vi "Actor Core.vi"(8 "error in":errorcluster, 11 "TranslationStageUI.lvclass":refnum<class "TranslationStageUI.lvclass">) -> (0 "error out":errorcluster, 3 "Actor out":refnum<class "Actor.lvclass">)   [LabVIEW 2023, in "TranslationStage_UI.lvlib" / "TranslationStageUI.lvclass"]
doc: "(<B>Filename</B>: Actor Framework.lvlib:Actor.lvclass:Actor Core.vi)\n\nReceives messages to the actor, reacts to them, and initiates any error handling that may shut the actor down.\n\nDescendant classes may override this VI to append parallel tasks for the actor to complete while it handles messages. Overrides use the Call Parent Class Method node."
uses:
  TranslationStageUI.lvclass
  <vilib>/ActorFramework/Actor/Actor.lvclass
  Scan_Data_For_Controller.ctl
  typedefs/TranslationStagePublicData.ctl
  <vilib>/ActorFramework/Actor/Actor.lvclass/Actor.ctl
  <vilib>/ActorFramework/Message Enqueuer/Message Enqueuer.lvclass/Message Enqueuer.ctl
  TranslationStageUI.lvclass/TranslationStageUI.ctl
  ConcreteClasses/ConcreteInstrumentClasses/KIM101/KIM101/KIM101.lvclass
  ConcreteClasses/ConcreteInstrumentClasses/Jiaxin_Stepper_Controller/Jiaxin_Stepper_Controller/Jiaxin_Stepper_Controller.lvclass
  Interfaces/InitDeinitInterface/InitDeinit Messages/Init Msg/Init Msg.lvclass/Init Msg.ctl
  Interfaces/AbstractInstrumentClasses/TranslationStages_LV/TranslationStagesInterface Messages/Goto Msg/Goto Msg.lvclass/Goto Msg.ctl
  Interfaces/AbstractInstrumentClasses/TranslationStages_LV/TranslationStagesInterface Messages/MoveBySteps Msg/MoveBySteps Msg.lvclass/MoveBySteps Msg.ctl
  SinglePhotonUI/Libraries/SPIController/SPIController Messages/InitScan Msg/InitScan Msg.lvclass/InitScan Msg.ctl
  SinglePhotonUI/Libraries/SPIController/SPIController Messages/StageMoved Msg/StageMoved Msg.lvclass/StageMoved Msg.ctl
  ConcreteClasses/ConcreteInstrumentClasses/Jiaxin_Stepper_Controller/Jiaxin_Stepper_Controller Messages/JX_GoHome Msg/JX_GoHome Msg.lvclass/JX_GoHome Msg.ctl
  <vilib>/ActorFramework/Message Enqueuer/Init from Existing Queue.vi
  <vilib>/ActorFramework/Message Enqueuer/Enqueue.vi
  Interfaces/InitDeinitInterface/InitDeinit Messages/Init Msg/Init Msg.lvclass
  <vilib>/ActorFramework/Stop Msg/Stop Msg.lvclass
  Interfaces/AbstractInstrumentClasses/TranslationStages_LV/TranslationStagesInterface Messages/Goto Msg/Goto Msg.lvclass
  Interfaces/AbstractInstrumentClasses/TranslationStages_LV/TranslationStagesInterface Messages/MoveBySteps Msg/MoveBySteps Msg.lvclass
  ConcreteClasses/ConcreteInstrumentClasses/Jiaxin_Stepper_Controller/Jiaxin_Stepper_Controller Messages/JX_SetHome Msg/JX_SetHome Msg.lvclass
  SinglePhotonUI/Libraries/SPIController/SPIController Messages/InitScan Msg/InitScan Msg.lvclass
  SinglePhotonUI/Libraries/SPIController/SPIController Messages/StageMoved Msg/StageMoved Msg.lvclass
  ConcreteClasses/ConcreteInstrumentClasses/Jiaxin_Stepper_Controller/Jiaxin_Stepper_Controller Messages/JX_GoHome Msg/JX_GoHome Msg.lvclass
  <vilib>/ActorFramework/Message Priority Queue/Priority Enqueue.vi
  <vilib>/ActorFramework/Message Enqueuer/Message Enqueuer.lvclass
  SinglePhotonUI/Libraries/SinglePhotonInterferenceUI/SinglePhotonInterferenceUI/SinglePhotonInterferenceUI.lvclass
  typedefs/typedefs.lvlib
  C:/Program Files/National Instruments/LabVIEW 2023/vi.lib/ActorFramework/Actor/Actor.lvclass
  C:/Users/quantum/Documents/LVDAQ/UIs/TranslationStage_UI/TranslationStage_UI/TranslationStageUI.lvclass
  C:/Users/quantum/Documents/LVDAQ/Interfaces/InitDeinitInterface/InitDeinitComm/InitDeinitComm.lvclass
  C:/Users/quantum/Documents/LVDAQ/Interfaces/AbstractInstrumentClasses/TranslationStages_LV/TranslationStagesComm/TranslationStagesComm.lvclass
  <vilib>/Utility/Data Type/NI_Data Type.lvlib
panel:
  out "value":variant
  in  "Go To":bool
  in  "Tab Control":T1(tab)
  in  "VISA resource name":refnum<visa-resource-name>
  in  "Control":enum16{"KIM", "Stepper Motors"}(ring)=enum."Stepper Motors"
  in  "Address":string="97102699"
  in  "Init motor":bool
  in  "Restart Piezo":bool
  in  "Exit":bool
  in  "Experiment Jog":i32(ring) caption="Experiment" items=["Imaging", "Interferometer"]
  in  "Jog Left HOM":bool
  in  "Jog Right HOM":bool
  in  "Jog Up":bool
  in  "Jog Left":bool
  in  "Jog Right":bool
  in  "Jog Down":bool
  in  "Jog Z Out":bool
  in  "Jog Z In":bool
  in  "Steps":i32(slide)=1 min=1 max=60000 step=1 scale=1.0..60000.0
  out "Position X":i32
  out "Position Z":i32
  out "Position Y":i32
  out "Position HOM":i32
  out "Scanning":bool
  in  "Get Measurements":bool
  in  "Steps Per Segment":i32=1 min=1 max=60000 step=1
  in  "Interferometer\nDirection":enum16{"Forward", "Backwards"}(ring)=enum."Backwards"
  in  "Focus Scan Direction":enum16{"Forward", "Backwards"}(ring)=enum."Backwards"
  in  "Y Scan Direction":enum16{"Forward", "Backwards"}(ring)=enum."Backwards"
  in  "Focus Steps":u32=1 min=1 max=60000 step=1
  in  "Y Pixels":u32=1 min=1 max=60000 step=1
  in  "X Pixels":u32=1 min=1 max=60000 step=1
  in  "Scan":bool
  in  "Acq Per Step":u8=1 min=1 step=1
  in  "X Scan Direction":enum16{"Forward", "Backwards"}(ring)=enum."Backwards"
  in  "Interferometer\nSegments":u32=1 min=1 max=60000 step=1
  in  "Experiment Scan":i32(ring) caption="Experiment" items=["Imaging", "Interferometer"]
  in  "HOM Channel":i32(ring)=1 items=["Channel0", "Channel1", "Channel2", "Channel3", "Channel4"]
  in  "Z Channel":i32(ring)=1 items=["Channel0", "Channel1", "Channel2", "Channel3", "Channel4"]
  in  "Y Channel":i32(ring)=1 items=["Channel0", "Channel1", "Channel2", "Channel3", "Channel4"]
  in  "X Channel":i32(ring)=1 items=["Channel0", "Channel1", "Channel2", "Channel3", "Channel4"]
  in  "Scan Data":T2
  in  "Scan Data":T2
  out "VI":refnum<vi>
  in  "Jog Parameters":T3={"JogAcceleration"=0, "JogStepFwd"=1, "JogMode"=1, "JogRate"=0, "JogStepRev"=1} {"JogStepRev" min=1 max=50000 step=1; "JogMode" items=["Continuous"=1, "Step"=2]; "JogStepFwd" min=1 max=100000 step=1}
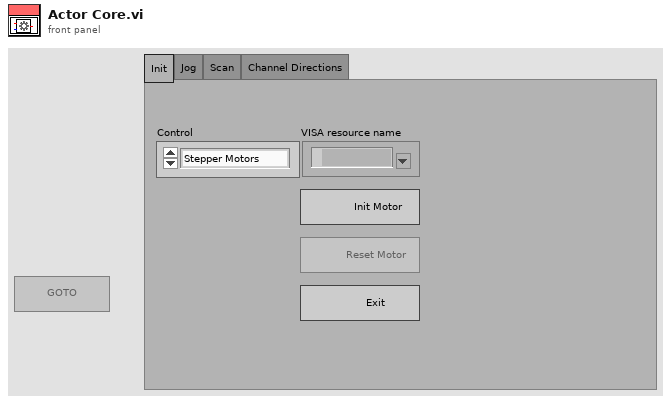
[diagram p1: front panel]
types:
  T1 = enum32{"Init", "Jog", "Scan", "Channel Directions"}
  T2 = typedef "typedefs.lvlib/Scan_Data_For_Controller.ctl" = cluster{"Scan Segments X":u32, "Scan Segments Y":u32, "Acq per step":u8, "Get Measurements?":bool}
  T3 = cluster{"JogAcceleration":i32, "JogStepFwd":i32, "JogMode":i32, "JogRate":i32, "JogStepRev":i32}
  T4 = typedef "typedefs.lvlib/TranslationStagePublicData.ctl" = cluster{"Scanning Instrument":bool, "Path":path, "FileName":string, "Scan Segments":u32, "Step Time (us)":u32, "Polarity":enum16{"Positive", "Negative"}, "Direction":enum16{"Forward", "Backwards"}, "Steps":u32, "Acq per step":u32, "First Scan Move?":bool, "Scan Segments X":u32, "Scan Segments Y":u32, "Position":i32, "Position 2":i32, "Position 3":i32, "Position 4":i32, "Home 1":i32, "Home 2":i32, "Home 3":i32, "Home 4":i32, "Going Home?":bool, "Selected Motor":enum16{"KIM", "Stepper Motors"}, "Scanning Motor":bool}
  T5 = enum8{"Enabled", "Disabled", "Disabled and Grayed Out"}
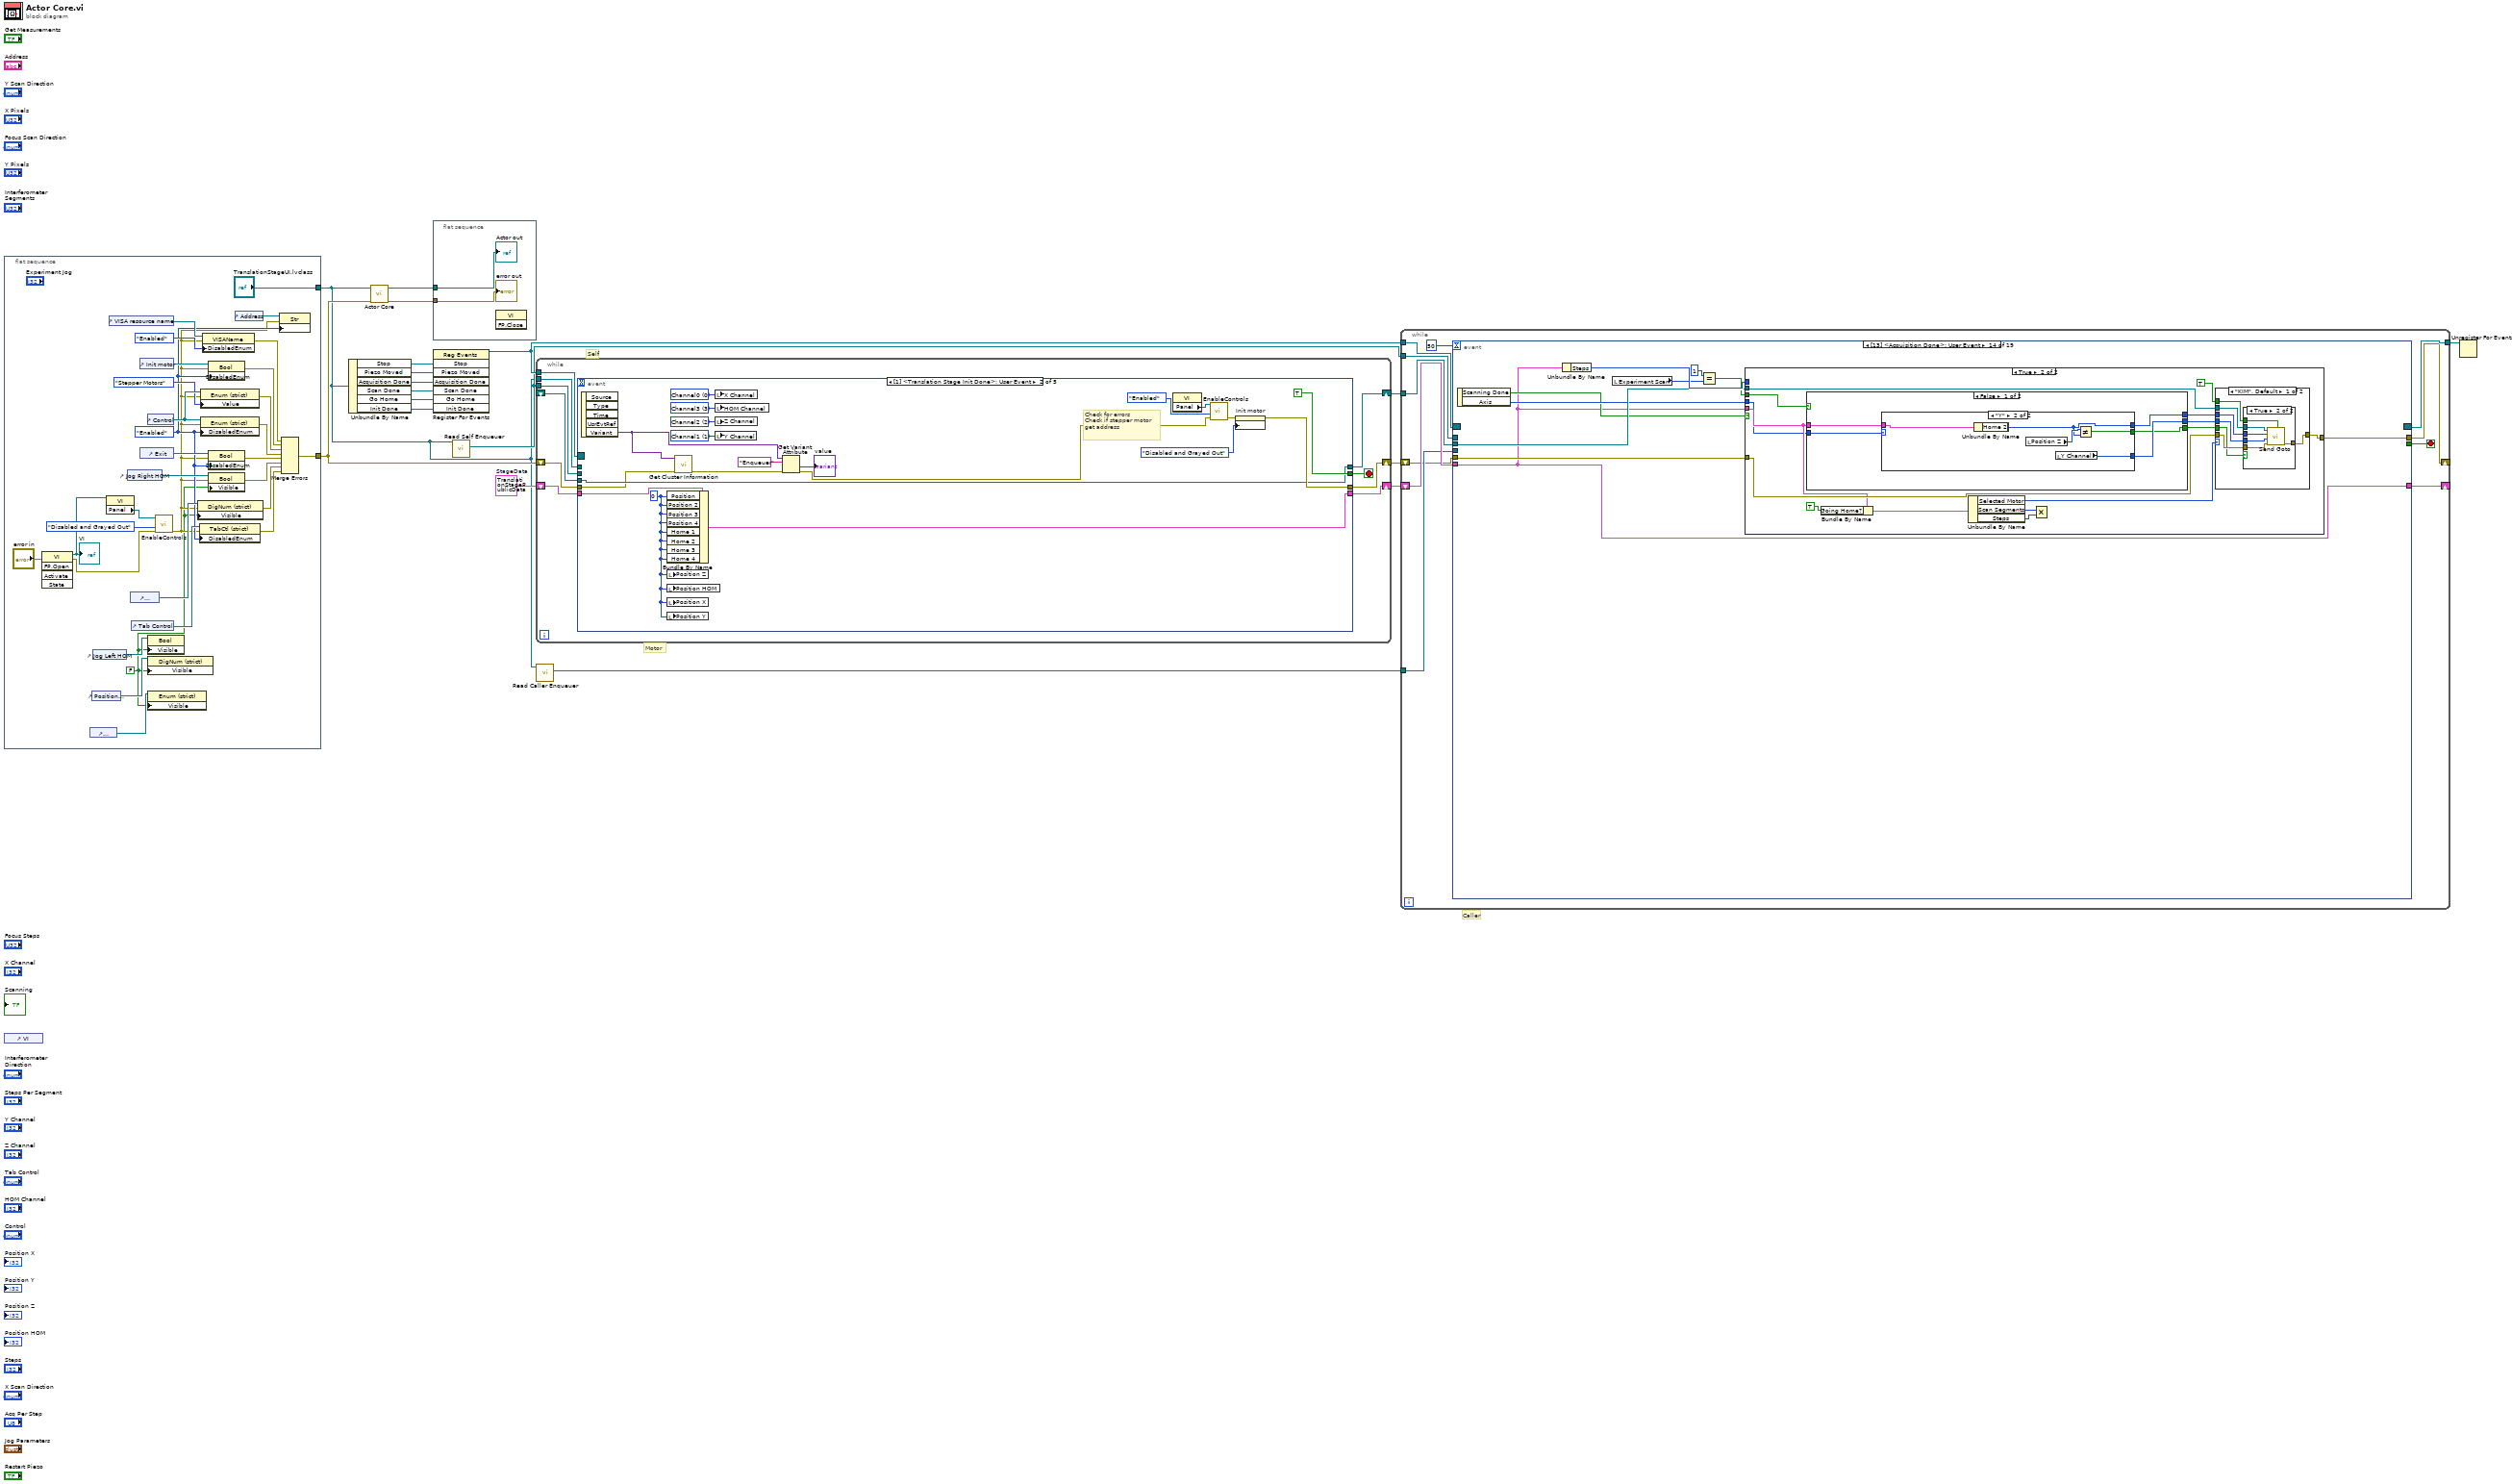
[diagram p0: block diagram]
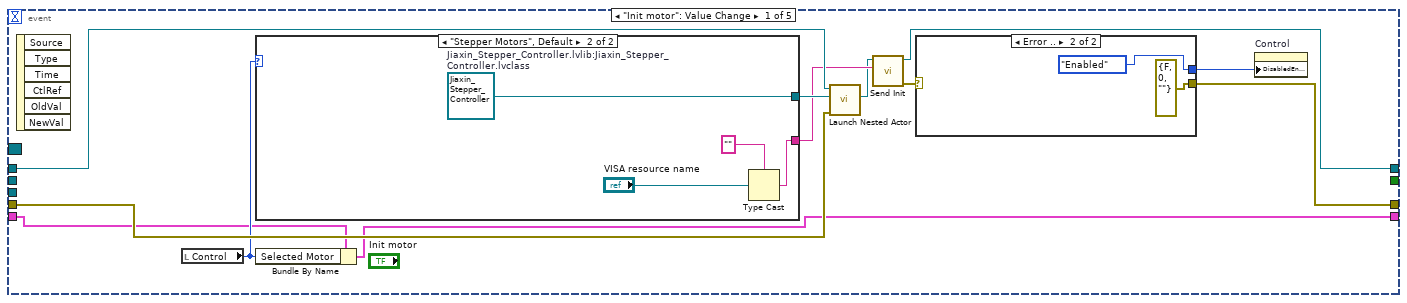
[diagram p2: hidden frame]
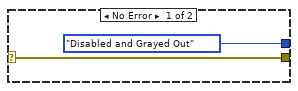
[diagram p3: hidden frame]
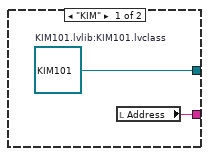
[diagram p4: hidden frame]
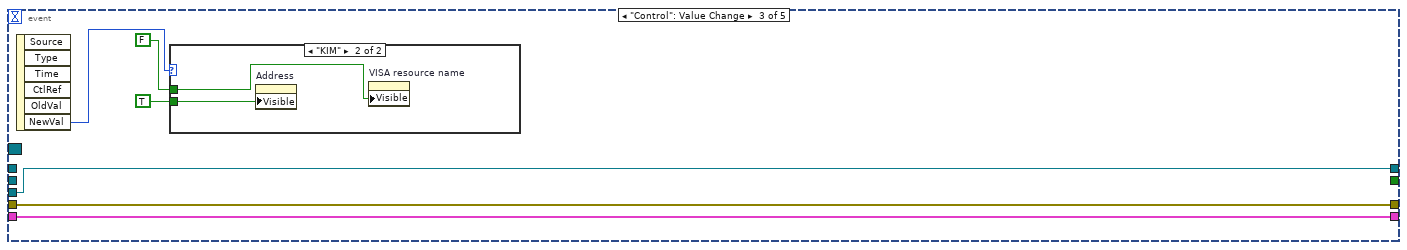
[diagram p5: hidden frame]
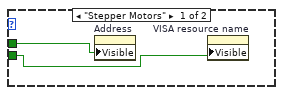
[diagram p6: hidden frame]
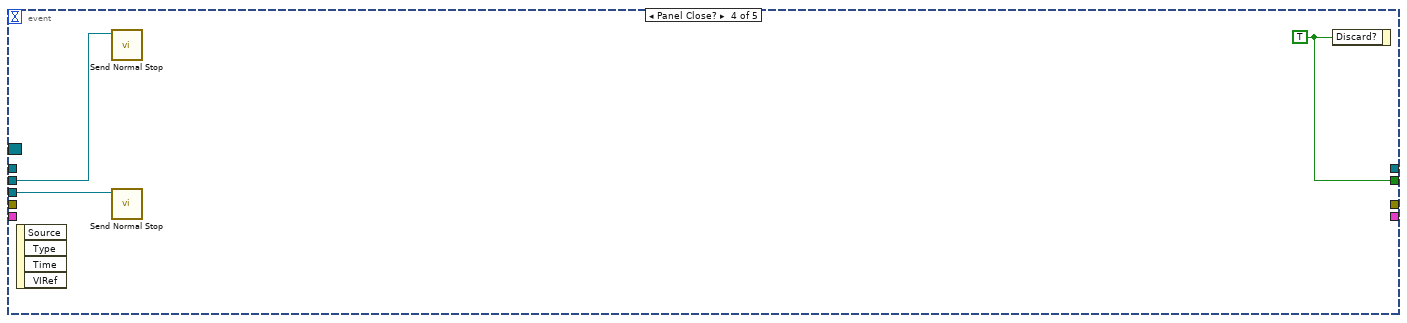
[diagram p7: hidden frame]
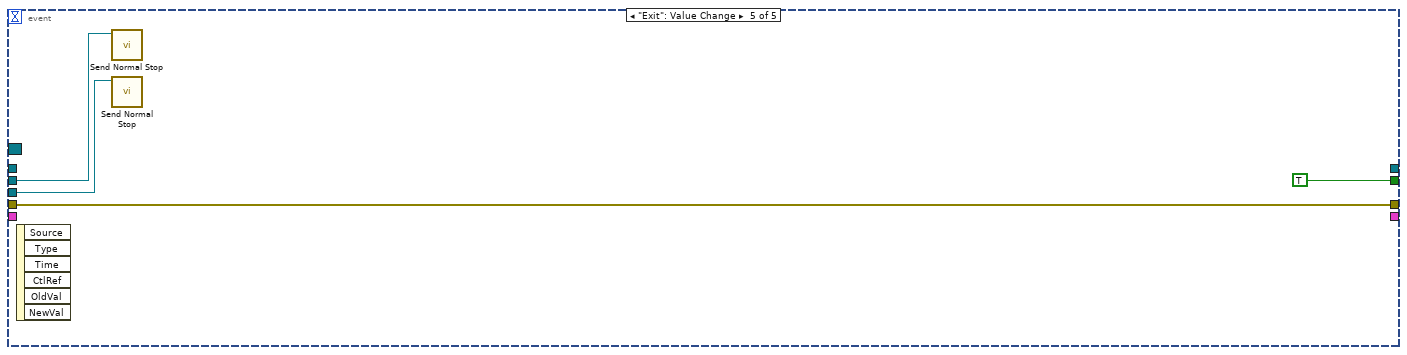
[diagram p8: hidden frame]
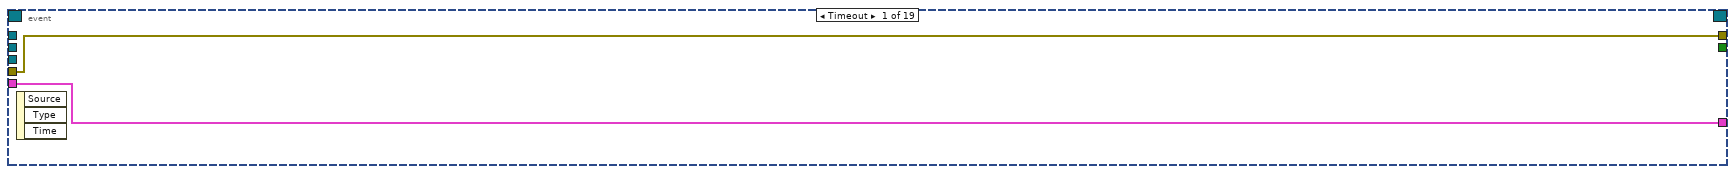
[diagram p9: hidden frame]
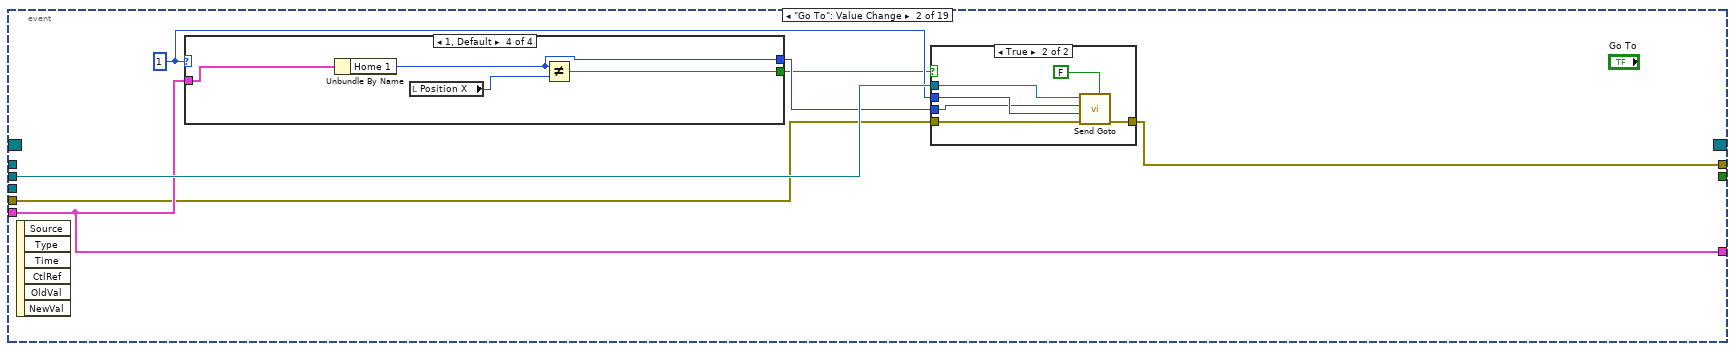
[diagram p10: hidden frame]
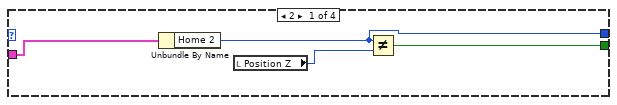
[diagram p12: hidden frame]
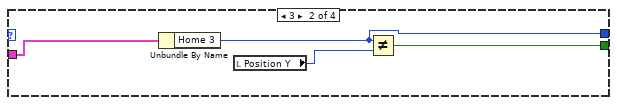
[diagram p13: hidden frame]
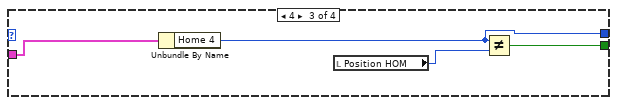
[diagram p14: hidden frame]
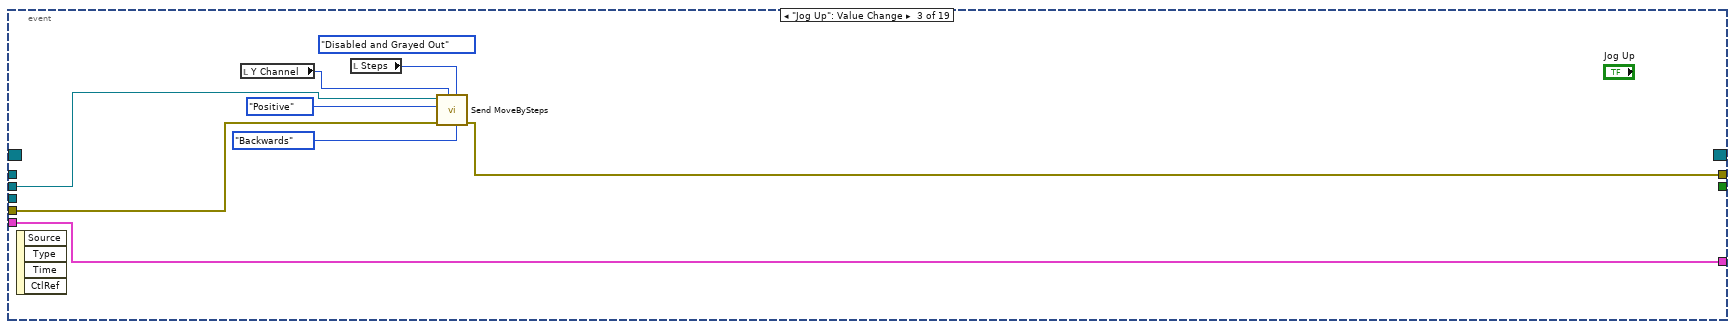
[diagram p15: hidden frame]
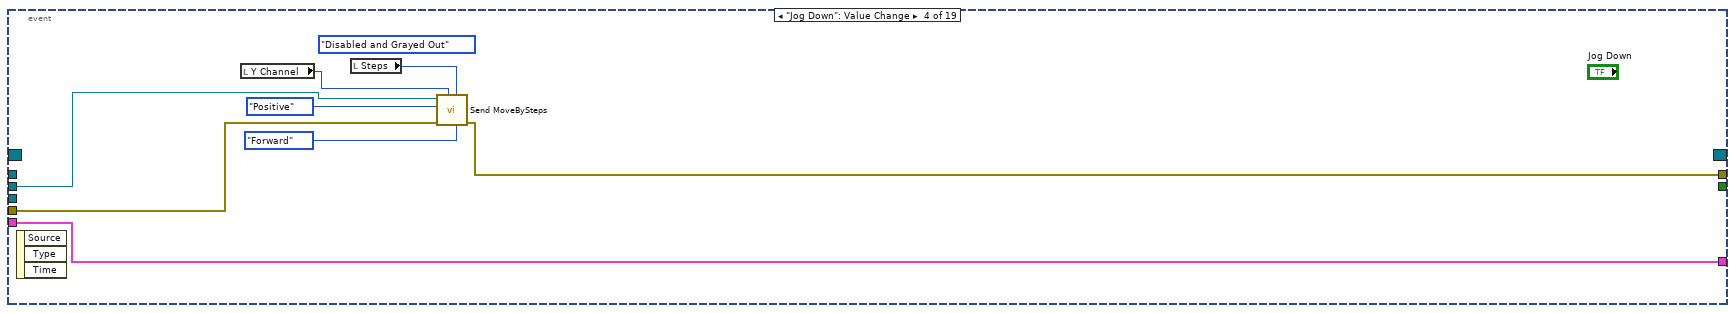
[diagram p16: hidden frame]
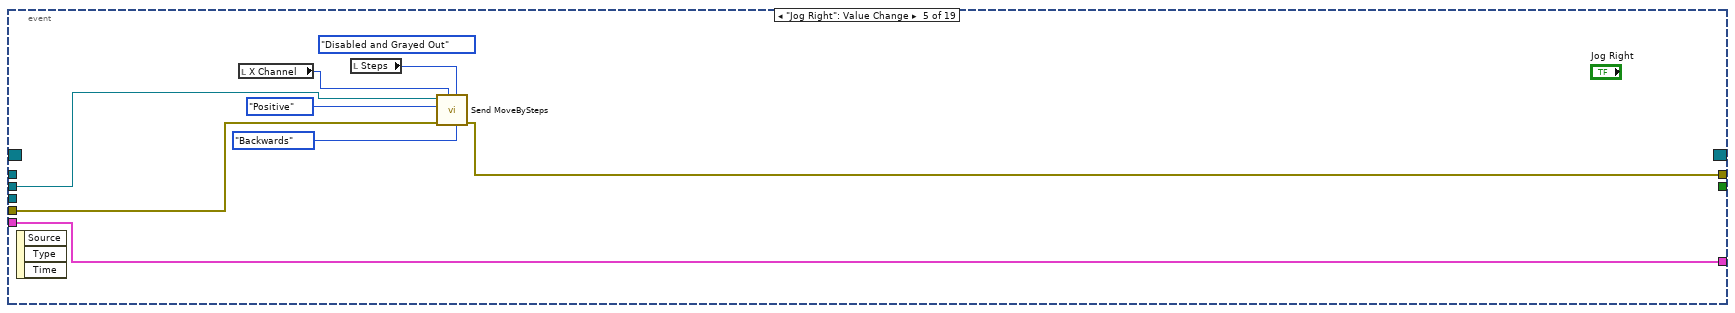
[diagram p17: hidden frame]
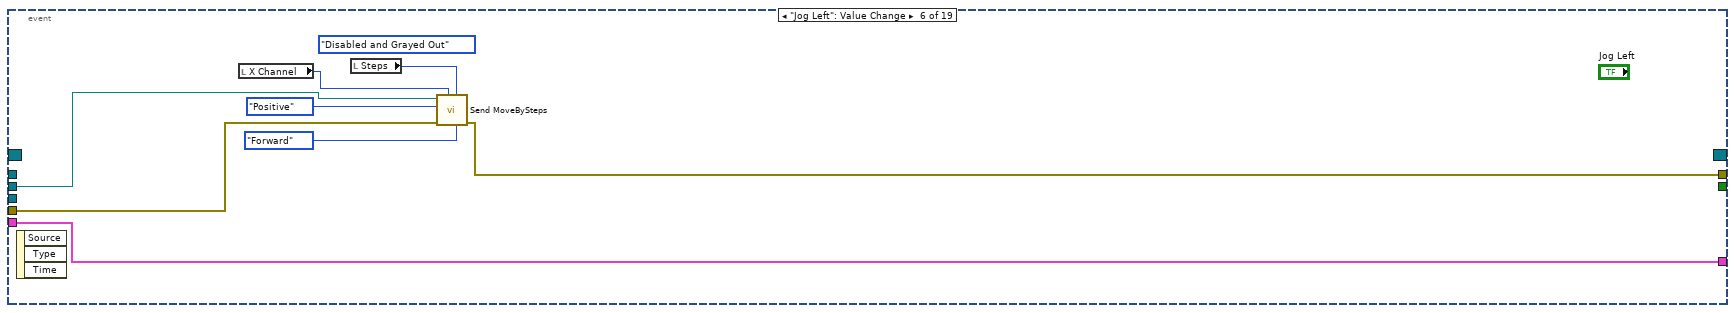
[diagram p18: hidden frame]
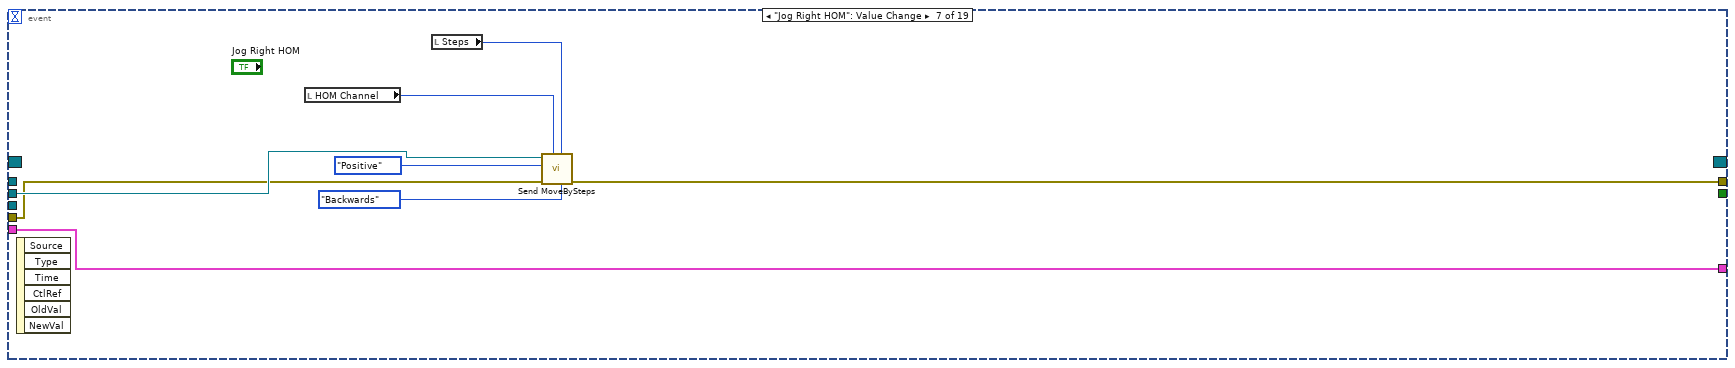
[diagram p19: hidden frame]
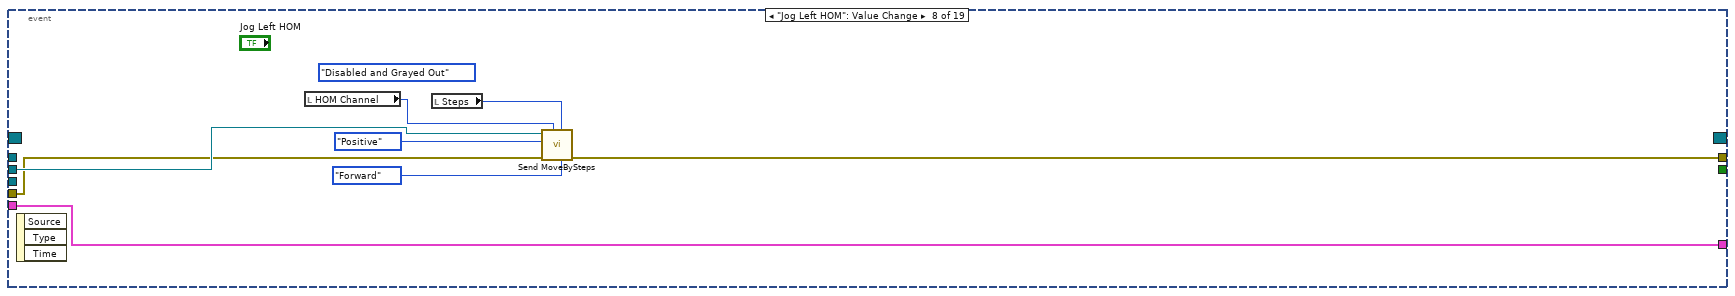
[diagram p20: hidden frame]
diagram:
  w5 = T4 {"Scanning Instrument"=FALSE, "Path"=path "", "FileName"="", "Scan Segments"=0, "Step Time (us)"=100, "Polarity"=enum."Positive", "Direction"=enum."Forward", "Steps"=1, "Acq per step"=1, "First Scan Move?"=FALSE, "Scan Segments X"=0, "Scan Segments Y"=0, "Position"=0, "Position 2"=0, "Position 3"=0, "Position 4"=0, "Home 1"=0, "Home 2"=0, "Home 3"=0, "Home 4"=0, "Going Home?"=FALSE, "Selected Motor"=enum."Stepper Motors", "Scanning Motor"=FALSE}  # StageData
  # "Motor"
  # "Self"
  # "Caller"
  n1 = flat-sequence {
    tunnel: ["TranslationStageUI.lvclass"] -> w2
    tunnel: [w34] -> w3
    frame #0 {
      w19 = FALSE ("Visible")
      w25 = T5."Enabled" ("Disabled")
      n2 = invoke class="VI" method="FP.Open"(error in="error in") -> (reference out=w47:refnum<vi>, error out=w45:errorcluster)  [unwired: 4 in, 3 out]
      "VI" <- w47
      n3 = control-ref of="Interferometer\nDirection"() -> (w20:refnum<vi>)
      n4 = control-ref of="Position HOM"() -> (w21:refnum<vi>)
      n5 = control-ref of="Jog Left HOM"() -> (w22:refnum<vi>)
      n6 = property class="VI"(reference=w47) -> ("Panel"=w46:refnum<vi>)  [unwired: 1 in, 2 out]
      n7 = control-ref of="VISA resource name"() -> (w36:refnum<vi>)
      n8 = control-ref of="Jog Right HOM"() -> (w42:refnum<vi>)
      n9 = control-ref of="Interferometer\nSegments"() -> (w40:refnum<vi>)
      n10 = control-ref of="Tab Control"() -> (w26:refnum<vi>)
      n11 = control-ref of="Init motor"() -> (w43:refnum<vi>)
      n12 = control-ref of="Exit"() -> (w41:refnum<vi>)
      n13 = control-ref of="Control"() -> (w38:refnum<vi>)
      n14 = property class="Bool"(reference=w22, "Visible"=w19) -> ()  [unwired: 1 in, 2 out]
      n15 = property class="DigNum (strict)"(reference=w21, "Visible"=w19) -> ()  [unwired: 1 in, 2 out]
      n16 = property class="Enum (strict)"(reference=w20, "Visible"=w19) -> ()  [unwired: 1 in, 2 out]
      n17 = call "EnableControls.vi"("error in (no error)"=w45, "Disabled"=T5."Disabled and Grayed Out", "Panel in"=w46) -> ("error out"=w24:errorcluster)  [unwired: 8 in]
      n18 = property class="DigNum (strict)"(reference=w40, error in=w24, "Visible"=w19) -> (error out=w27:errorcluster)  [unwired: 1 out]
      n19 = property class="TabCtl (strict)"(reference=w26, error in=w24, "DisabledEnum"=w25) -> (error out=w23:errorcluster)  [unwired: 1 out]
      n20 = property class="Enum (strict)"(reference=w38, error in=w24, "Value"=enum16{"KIM", "Stepper Motors"}."Stepper Motors") -> (error out=w30:errorcluster)  [unwired: 1 out]
      n21 = property class="Enum (strict)"(reference=w38, error in=w24, "DisabledEnum"=w25) -> (error out=w31:errorcluster)  [unwired: 1 out]
      n22 = property class="VISAName"(reference=w36, error in=w24, "DisabledEnum"=T5."Enabled" ("Disabled")) -> (error out=w28:errorcluster)  [unwired: 1 out]
      n23 = property class="Bool"(reference=w43, error in=w24, "DisabledEnum"=w25) -> (error out=w29:errorcluster)  [unwired: 1 out]
      n24 = property class="Bool"(reference=w41, error in=w24, "DisabledEnum"=w25) -> (error out=w32:errorcluster)  [unwired: 1 out]
      n25 = property class="Bool"(reference=w42, error in=w24, "Visible"=w19) -> (error out=w33:errorcluster)  [unwired: 1 out]
      n26 = control-ref of="Address"() -> (w39:refnum<vi>)
      n27 = property class="Str"(reference=w39, error in=w24, "DisabledEnum"=w25) -> ()  [unwired: 2 out]
      n28 = Merge Errors(w28, w29, w30, w31, w32, w33, w27, w23) -> (w34:errorcluster)
    }
  }
  n29 = control-ref of="VI"() -> ()  [unwired: 1 out]
  n30 = Unbundle By Name(w2) -> ("Stop"=w15:refnum<user-event>, "Piezo Moved"=w14:refnum<user-event>, "Acquisition Done"=w10:refnum<user-event>, "Scan Done"=w9:refnum<user-event>, "Go Home"=w8:refnum<user-event>, "Init Done"=w1:refnum<user-event>)
  n31 = call-parent "Actor Core.vi"("error in"=w3, "Actor in"=w2) -> ("error out"=w18:errorcluster, "Actor out"=w17:refnum<class "Actor.lvclass">)  [unwired: 8 in]
  n32 = flat-sequence {
    tunnel: w18 -> [w51]
    tunnel: w17 -> [w50]
    frame #0 {
      n33 = invoke class="VI" method="FP.Close"() -> ()  [unwired: 3 in, 3 out]
      "error out" <- w51
      "Actor out" <- w50
    }
  }
  n34 = register-events(w15, w14, w10, w9, w8, w1) -> (reference out=w7:refnum<event-registration>)  [unwired: 2 in, 1 out]
  n35 = call <vilib>:"Read Self Enqueuer.vi"("Actor"=w2) -> ("Self Enqueuer"=w4:refnum<class "Message Enqueuer.lvclass">)  [unwired: 10 in]
  n36 = while {
    tunnel: w2 -> [w54]
    shift-right: [w56] -> w11
    shift-left: w3 -> [w58]
    tunnel: w7 -> [w61]
    shift-right: [w60] -> w6
    shift-left: w5 -> [w59]
    shift-right: [w57] -> w16
    shift-left: _ -> [w55]
    tunnel: w4 -> [w52]
    stop <- w53 stop-if-true
    n37 = event shown="[1] <Translation Stage Init Done>: User Event" {
      selector: w61 -> [_ _ _ _ _]
      dyn-events: _ -> [_ _ _ _ _]
      timeout: _ -> [_ _ _ _ _]
      tunnel: [w69 w99 w106 _ _] -> w60
      tunnel: w59 -> [w70 w98 w106 _ _]
      tunnel: w58 -> [w73 w89 w105 _ w118]
      tunnel: [w68 w97 w105 _ w118] -> w56
      tunnel: [w63 w95 w104 _ _] -> w57
      tunnel: w55 -> [_ w95 w104 w116 w120]
      tunnel: w54 -> [w72 _ _ _ _]
      tunnel: [_ TRUE _ w114 TRUE] -> w53
      tunnel: w52 -> [_ _ _ w115 w119]
      event "Init motor": Value Change {
        n38 = event-data() -> ()  [unwired: 1 in, 6 out]
        n39 = local read "Control"() -> (w71:enum16{"KIM", "Stepper Motors"})
        n40 = case shown="\"Stepper Motors\", Default" w71 {
          tunnel: [w78 w81] -> w66
          tunnel: [w79 w80] -> w65
          frame "KIM" {
            w78 = refnum<class "KIM101.lvclass"> refnum  # KIM101.lvlib:KIM101.lvclass
            n41 = local read "Address"() -> (w79:string)
          }
          frame "Stepper Motors", Default {
            w81 = refnum<class "Jiaxin_Stepper_Controller.lvclass"> refnum  # Jiaxin_Stepper_Controller.lvlib:Jiaxin_Stepper_Controller.lvclass
            n42 = Type Cast(type="" ("*(type *) &x"), x="VISA resource name") -> (*(type *) &x=w80:string)
          }
        }
        n43 = Bundle By Name(cluster=w70, "Selected Motor"=w71) -> (w69:T4)
        n44 = call <vilib>:"Launch Nested Actor.vi"("error in (no error)"=w73, "Nested Actor"=w66, "Caller Actor in"=w72) -> ("Nested Actor's Enqueuer"=w62:refnum<class "Message Enqueuer.lvclass">)  [unwired: 6 in, 2 out]
        n45 = call "Send Init.vi"("Address"=w65, "Message Enqueuer"=w62) -> ("error out"=w64:errorcluster, "Message Enqueuer out"=w63:refnum<class "Message Enqueuer.lvclass">)  [unwired: 8 in]
        n46 = case shown="Error .." w64 {
          selector: w64 -> [w75 _]
          tunnel: [w75 errorcluster {"status"=FALSE, "code"=0, "source"=""} ("error IO")] -> w68
          tunnel: [T5."Disabled and Grayed Out" ("Disabled") T5."Enabled" ("Disabled")] -> w67
          frame No Error {
          }
          frame Error {
          }
        }
        n47 = property on="Control" class="Enum (strict)"("DisabledEnum"=w67) -> ()  [unwired: 2 in, 2 out]
      }
      event User Event {
        w90 = 0
        w94 = 2 items=["Channel0", "Channel1", "Channel2", "Channel3", "Channel4"] ("Z Channel")
        w93 = 1 items=["Channel0", "Channel1", "Channel2", "Channel3", "Channel4"] ("Y Channel")
        w92 = 0 items=["Channel0", "Channel1", "Channel2", "Channel3", "Channel4"] ("X Channel")
        w91 = 3 items=["Channel0", "Channel1", "Channel2", "Channel3", "Channel4"] ("HOM Channel")
        # "Check for errors\nCheck if stepper motor\nget address"
        n48 = event-data() -> ("Variant"=w86:variant)  [unwired: 1 in, 4 out]
        n49 = Bundle By Name(cluster=w98, "Position"=w90, "Position 2"=w90, "Position 3"=w90, "Position 4"=w90, "Home 1"=w90, "Home 2"=w90, "Home 3"=w90, "Home 4"=w90) -> (w99:T4)
        n50 = local write "Position Z"(w90) -> ()
        n51 = local write "Position HOM"(w90) -> ()
        n52 = local write "Position X"(w90) -> ()
        n53 = local write "Position Y"(w90) -> ()
        n54 = call <vilib>:"Get Cluster Information.vi"("error in (no error)"=w89, "variant"=w86) -> ("error out"=w88:errorcluster)  [unwired: 8 in, 1 out]
        n55 = local write "X Channel"(w92) -> ()
        n56 = local write "HOM Channel"(w91) -> ()
        n57 = local write "Z Channel"(w94) -> ()
        n58 = local write "Y Channel"(w93) -> ()
        n59 = Get Variant Attribute(Variant=w86, name="Enqueuer", error in=w88) -> (value=→"value":variant, error out=w87:errorcluster)  [unwired: 1 in, 2 out]
        n60 = property class="VI"() -> ("Panel"=w101:refnum<vi>)  [unwired: 2 in, 2 out]
        n61 = call "EnableControls.vi"("error in (no error)"=w87, "Disabled"=T5."Enabled", "Panel in"=w101) -> ("error out"=w103:errorcluster)  [unwired: 8 in]
        n62 = property on="Init motor" class="Bool"(error in=w103, "DisabledEnum"=T5."Disabled and Grayed Out" ("Disabled")) -> (error out=w97:errorcluster)  [unwired: 1 in, 1 out]
      }
      event "Control": Value Change {
        n63 = event-data() -> ("NewVal"=w107:enum16{"KIM", "Stepper Motors"})  [unwired: 1 in, 5 out]
        n64 = case shown="\"KIM\"" w107 {
          tunnel: FALSE ("Visible") -> [w111 w112]
          tunnel: TRUE ("Visible") -> [w110 w113]
          frame "Stepper Motors" {
            n65 = property on="Address" class="Str"("Visible"=w111) -> ()  [unwired: 2 in, 2 out]
            n66 = property on="VISA resource name" class="VISAName"("Visible"=w110) -> ()  [unwired: 2 in, 2 out]
          }
          frame "KIM" {
            n67 = property on="Address" class="Str"("Visible"=w113) -> ()  [unwired: 2 in, 2 out]
            n68 = property on="VISA resource name" class="VISAName"("Visible"=w112) -> ()  [unwired: 2 in, 2 out]
          }
        }
      }
      event Panel Close? {
        w114 = TRUE ("Discard?")
        n69 = event-data() -> ()  [unwired: 1 in, 4 out]
        n70 = call <vilib>:"Send Normal Stop.vi"("Message Enqueuer"=w115) -> ()  [unwired: 10 in, 1 out]
        n71 = call <vilib>:"Send Normal Stop.vi"("Message Enqueuer"=w116) -> ()  [unwired: 10 in, 1 out]
        n72 = event-data("Discard?"=w114) -> ()  [unwired: 1 in, 1 out]
      }
      event "Exit": Value Change {
        n73 = event-data() -> ()  [unwired: 1 in, 6 out]
        n74 = call <vilib>:"Send Normal Stop.vi"("Message Enqueuer"=w119) -> ()  [unwired: 10 in, 1 out]
        n75 = call <vilib>:"Send Normal Stop.vi"("Message Enqueuer"=w120) -> ()  [unwired: 10 in, 1 out]
      }
    }
  }
  n76 = call <vilib>:"Read Caller Enqueuer.vi"("Actor"=w2) -> ("Caller Enqueuer"=w12:refnum<class "Message Enqueuer.lvclass">)  [unwired: 10 in]
  n77 = while {
    tunnel: w16 -> [w130]
    tunnel: w7 -> [w131]
    tunnel: [w128] -> w13
    tunnel: w4 -> [w127]
    shift-right: [w125] -> _
    shift-left: w6 -> [w126]
    tunnel: w12 -> [w124]
    shift-right: [w122] -> _
    shift-left: w11 -> [w123]
    stop <- w129 stop-if-true
    n78 = event shown="[13] <Acquisition Done>: User Event" {
      selector: w131 -> [_ _ _ _ _ _ _ _ _ _ _ _ _ _ _ _ _ _ _]
      dyn-events: [_ _ _ _ _ _ _ _ _ _ _ _ _ _ _ _ _ _ _] -> w128
      timeout: 50 -> [_ _ _ _ _ _ _ _ _ _ _ _ _ _ _ _ _ _ _]
      tunnel: w130 -> [_ w140 w171 w179 w187 w195 w203 w211 w219 w227 w233 w246 _ w320 _ w425 _ w450 w454]
      tunnel: [_ _ _ _ _ _ _ _ _ _ _ _ _ _ _ _ TRUE _ _] -> w129
      tunnel: w127 -> [_ _ _ _ _ _ _ _ _ _ _ _ _ _ _ _ _ w449 w453]
      tunnel: w126 -> [w132 w139 w165 w173 w181 w189 w197 w205 w213 w221 w231 w254 w309 w314 w403 w437 w445 w448 w452]
      tunnel: [w132 w139 w165 w173 w181 w189 w197 w205 w213 w221 w231 w269 w309 w314 w408 w436 w445 w448 w452] -> w125
      tunnel: w124 -> [_ _ _ _ _ _ _ _ _ _ _ w265 _ _ w411 _ _ _ _]
      tunnel: w123 -> [w133 w137 w170 w178 w186 w194 w202 w210 w218 w226 w232 w255 w308 w323 w409 w424 w444 w447 w451]
      tunnel: [w133 w136 w169 w177 w185 w193 w201 w209 w217 w225 w228 w257 w308 w322 w410 w428 w444 w447 w451] -> w122
      event Timeout {
        n79 = event-data() -> ()  [unwired: 1 in, 3 out]
      }
      event "Go To": Value Change {
        w135 = 1 ("Channel")
        n80 = event-data() -> ()  [unwired: 1 in, 6 out]
        n81 = case shown="1, Default" w135 {
          tunnel: w139 -> [w151 w155 w159 w163]
          tunnel: [w148 w152 w157 w161] -> w138
          tunnel: [w149 w153 w156 w160] -> w134
          frame 2 {
            n82 = Unbundle By Name(w151) -> ("Home 2"=w148:i32)
            n83 = local read "Position Z"() -> (w150:i32)
            n84 = Not Equal?(x=w148, y=w150) -> (x != y?=w149:bool)
          }
          frame 3 {
            n85 = Unbundle By Name(w155) -> ("Home 3"=w152:i32)
            n86 = local read "Position Y"() -> (w154:i32)
            n87 = Not Equal?(x=w152, y=w154) -> (x != y?=w153:bool)
          }
          frame 4 {
            n88 = Unbundle By Name(w159) -> ("Home 4"=w157:i32)
            n89 = local read "Position HOM"() -> (w158:i32)
            n90 = Not Equal?(x=w157, y=w158) -> (x != y?=w156:bool)
          }
          frame 1, Default {
            n91 = Unbundle By Name(w163) -> ("Home 1"=w161:i32)
            n92 = local read "Position X"() -> (w162:i32)
            n93 = Not Equal?(x=w161, y=w162) -> (x != y?=w160:bool)
          }
        }
        n94 = case shown="True" w134 {
          tunnel: w140 -> [_ w147]
          tunnel: w138 -> [_ w143]
          tunnel: w137 -> [w141 w145]
          tunnel: [w141 w146] -> w136
          tunnel: w135 -> [_ w144]
          frame False {
          }
          frame True {
            n95 = call "Send Goto.vi"("Home?"=FALSE, "error in (no error)"=w145, "channel"=w144, "New Position"=w143, "Message Enqueuer"=w147) -> ("error out"=w146:errorcluster)  [unwired: 5 in, 1 out]
          }
        }
      }
      event "Jog Up": Value Change {
        (unwired) T5."Disabled and Grayed Out" ("Disabled")
        n96 = event-data() -> ()  [unwired: 1 in, 4 out]
        n97 = local read "Y Channel"() -> (w167:i32)
        n98 = local read "Steps"() -> (w166:i32)
        n99 = call "Send MoveBySteps.vi"("Direction"=enum16{"Forward", "Backwards"}."Backwards", "Steps"=w166, "Message Priority (Normal)"=w167, "error in (no error)"=w170, "Polarity"=enum16{"Positive", "Negative"}."Positive", "Message Enqueuer"=w171) -> ("error out"=w169:errorcluster)  [unwired: 4 in, 1 out]
      }
      event "Jog Down": Value Change {
        (unwired) T5."Disabled and Grayed Out" ("Disabled")
        n100 = event-data() -> ()  [unwired: 1 in, 3 out]
        n101 = local read "Y Channel"() -> (w175:i32)
        n102 = local read "Steps"() -> (w174:i32)
        n103 = call "Send MoveBySteps.vi"("Direction"=enum16{"Forward", "Backwards"}."Forward", "Steps"=w174, "Message Priority (Normal)"=w175, "error in (no error)"=w178, "Polarity"=enum16{"Positive", "Negative"}."Positive", "Message Enqueuer"=w179) -> ("error out"=w177:errorcluster)  [unwired: 4 in, 1 out]
      }
      event "Jog Right": Value Change {
        (unwired) T5."Disabled and Grayed Out" ("Disabled")
        n104 = event-data() -> ()  [unwired: 1 in, 3 out]
        n105 = local read "X Channel"() -> (w183:i32)
        n106 = local read "Steps"() -> (w182:i32)
        n107 = call "Send MoveBySteps.vi"("Direction"=enum16{"Forward", "Backwards"}."Backwards", "Steps"=w182, "Message Priority (Normal)"=w183, "error in (no error)"=w186, "Polarity"=enum16{"Positive", "Negative"}."Positive", "Message Enqueuer"=w187) -> ("error out"=w185:errorcluster)  [unwired: 4 in, 1 out]
      }
      event "Jog Left": Value Change {
        (unwired) T5."Disabled and Grayed Out" ("Disabled")
        n108 = event-data() -> ()  [unwired: 1 in, 3 out]
        n109 = local read "X Channel"() -> (w191:i32)
        n110 = local read "Steps"() -> (w190:i32)
        n111 = call "Send MoveBySteps.vi"("Direction"=enum16{"Forward", "Backwards"}."Forward", "Steps"=w190, "Message Priority (Normal)"=w191, "error in (no error)"=w194, "Polarity"=enum16{"Positive", "Negative"}."Positive", "Message Enqueuer"=w195) -> ("error out"=w193:errorcluster)  [unwired: 4 in, 1 out]
      }
      event "Jog Right HOM": Value Change {
        n112 = event-data() -> ()  [unwired: 1 in, 6 out]
        n113 = local read "HOM Channel"() -> (w199:i32)
        n114 = local read "Steps"() -> (w198:i32)
        n115 = call "Send MoveBySteps.vi"("Direction"=enum16{"Forward", "Backwards"}."Backwards", "Steps"=w198, "Message Priority (Normal)"=w199, "error in (no error)"=w202, "Polarity"=enum16{"Positive", "Negative"}."Positive", "Message Enqueuer"=w203) -> ("error out"=w201:errorcluster)  [unwired: 4 in, 1 out]
      }
      event "Jog Left HOM": Value Change {
        (unwired) T5."Disabled and Grayed Out" ("Disabled")
        n116 = event-data() -> ()  [unwired: 1 in, 3 out]
        n117 = local read "HOM Channel"() -> (w207:i32)
        n118 = local read "Steps"() -> (w206:i32)
        n119 = call "Send MoveBySteps.vi"("Direction"=enum16{"Forward", "Backwards"}."Forward", "Steps"=w206, "Message Priority (Normal)"=w207, "error in (no error)"=w210, "Polarity"=enum16{"Positive", "Negative"}."Positive", "Message Enqueuer"=w211) -> ("error out"=w209:errorcluster)  [unwired: 4 in, 1 out]
      }
      event "Jog Z Out": Value Change {
        (unwired) T5."Disabled and Grayed Out" ("Disabled")
        n120 = event-data() -> ()  [unwired: 1 in, 3 out]
        n121 = local read "Z Channel"() -> (w215:i32)
        n122 = local read "Steps"() -> (w214:i32)
        n123 = call "Send MoveBySteps.vi"("Direction"=enum16{"Forward", "Backwards"}."Backwards", "Steps"=w214, "Message Priority (Normal)"=w215, "error in (no error)"=w218, "Polarity"=enum16{"Positive", "Negative"}."Positive", "Message Enqueuer"=w219) -> ("error out"=w217:errorcluster)  [unwired: 4 in, 1 out]
      }
      event "Jog Z In": Value Change {
        n124 = event-data() -> ()  [unwired: 1 in, 3 out]
        n125 = local read "Z Channel"() -> (w223:i32)
        n126 = local read "Steps"() -> (w222:i32)
        n127 = call "Send MoveBySteps.vi"("Direction"=enum16{"Forward", "Backwards"}."Forward", "Steps"=w222, "Message Priority (Normal)"=w223, "error in (no error)"=w226, "Polarity"=enum16{"Positive", "Negative"}."Positive", "Message Enqueuer"=w227) -> ("error out"=w225:errorcluster)  [unwired: 4 in, 1 out]
      }
      event "Restart Piezo": Value Change {
        n128 = event-data() -> ()  [unwired: 1 in, 3 out]
        n129 = Unbundle By Name(w231) -> ("Selected Motor"=w230:enum16{"KIM", "Stepper Motors"})
        n130 = case shown="\"KIM\", Default" w230 {
          tunnel: [w234 w237] -> w229
          frame "Stepper Motors" {
            n131 = local read "VISA resource name"() -> (w235:refnum<visa-resource-name>)
            n132 = Type Cast(type="" ("*(type *) &x"), x=w235) -> (*(type *) &x=w234:string)
          }
          frame "KIM", Default {
            n133 = local read "Address"() -> (w237:string)
          }
        }
        n134 = call "Send Init.vi"("error in (no error)"=w232, "Address"=w229, "Message Enqueuer"=w233) -> ("error out"=w228:errorcluster)  [unwired: 7 in, 1 out]
      }
      event "Scan": Value Change {
        n135 = event-data() -> ()  [unwired: 1 in, 3 out]
        n136 = local write "Scanning"(TRUE ("Scanning")) -> ()
        n137 = local read "Get Measurements"() -> (w243:bool)
        n138 = property on="Restart Piezo" class="Bool"(error in=w255, "DisabledEnum"=T5."Enabled" ("Disabled")) -> (error out=w245:errorcluster)  [unwired: 1 in, 1 out]
        n139 = local read "Interferometer\nSegments"() -> (w248:u32)
        n140 = property on="Scan" class="Bool"(error in=w255, "DisabledEnum"=T5."Disabled" ("Disabled")) -> (error out=w258:errorcluster)  [unwired: 1 in, 1 out]
        n141 = local read "Experiment Scan"() -> (w249:i32)
        n142 = local read "Acq Per Step"() -> (w260:u8)
        n143 = local read "X Pixels"() -> (w262:u32)
        n144 = local read "Y Pixels"() -> (w261:u32)
        n145 = Select(t=TRUE, s=w243, f=FALSE) -> (s? t:f=w240:bool)
        n146 = local read "Interferometer\nDirection"() -> (w268:enum16{"Forward", "Backwards"})
        n147 = local read "Steps Per Segment"() -> (w247:i32)
        n148 = case shown="0, Default" w249 {
          tunnel: w262 -> [_ w287]
          tunnel: w261 -> [_ w286]
          tunnel: [w278 w284] -> w259
          tunnel: w248 -> [w276 _]
          tunnel: w260 -> [w275 w285]
          tunnel: w246 -> [w273 w281]
          tunnel: w245 -> [w272 w280]
          tunnel: [w271 w279] -> w244
          tunnel: w243 -> [w270 w282]
          frame 1 {
            n149 = call "Send JX_SetHome.vi"("error in (no error)"=w272, "Message Enqueuer"=w273) -> ("error out"=w271:errorcluster)  [unwired: 8 in, 1 out]
            n150 = Bundle By Name(cluster="Scan Data", "Scan Segments X"=w276, "Scan Segments Y"=u32 0, "Acq per step"=w275, "Get Measurements?"=w270) -> (w278:T2)
          }
          frame 0, Default {
            n151 = call "Send JX_SetHome.vi"("error in (no error)"=w280, "Message Enqueuer"=w281) -> ("error out"=w279:errorcluster)  [unwired: 8 in, 1 out]
            n152 = Bundle By Name(cluster="Scan Data", "Scan Segments X"=w287, "Scan Segments Y"=w286, "Acq per step"=w285, "Get Measurements?"=w282) -> (w284:T2)
          }
        }
        n153 = Unbundle By Name(w254) -> ("Position"=w253:i32, "Position 2"=w252:i32, "Position 3"=w251:i32, "Position 4"=w250:i32)
        n154 = Not(x=w240) -> (.not. x?=w239:bool)
        n155 = Bundle By Name(cluster=w254, "First Scan Move?"=w240, "Scanning Instrument"=w240, "Scanning Motor"=w239, "Scan Segments"=w248, "Direction"=w268, "Steps"=w247, "Acq per step"=w260, "Scan Segments X"=w262, "Scan Segments Y"=w261, "Polarity"=enum16{"Positive", "Negative"}."Positive", "Step Time (us)"=u32 0 ("Speed"), "Home 1"=w253, "Home 2"=w252, "Home 3"=w251, "Home 4"=w250) -> (w269:T4)
        n156 = call "Send InitScan.vi"("error in (no error)"=w255, "event data"=w259, "Message Enqueuer"=w265) -> ("error out"=w256:errorcluster)  [unwired: 7 in, 1 out]
        n157 = Merge Errors(w256, w244, w258) -> (w257:errorcluster)
      }
      event "Experiment Jog", "Experiment Scan": Value Change {
        n158 = event-data() -> ("NewVal"=w288:i32)  [unwired: 1 in, 5 out]
        n159 = local write "Experiment Scan"(w288) -> ()
        n160 = case shown="0, Default" w288 {
          tunnel: [TRUE ("Visible") FALSE ("Visible")] -> w291
          tunnel: [w310 w312] -> w289
          tunnel: [w310 w312] -> w302
          frame 0, Default {
            w310 = FALSE ("Visible")
          }
          frame 1 {
            w312 = TRUE ("Visible")
          }
        }
        n161 = local write "Experiment Jog"(w288) -> ()
        n162 = control-ref of="Focus Scan Direction"() -> (w306:refnum<vi>)
        n163 = control-ref of="X Scan Direction"() -> (w304:refnum<vi>)
        n164 = control-ref of="Y Scan Direction"() -> (w305:refnum<vi>)
        n165 = control-ref of="Jog Right HOM"() -> (w290:refnum<vi>)
        n166 = control-ref of="Interferometer\nDirection"() -> (w307:refnum<vi>)
        n167 = control-ref of="Interferometer\nSegments"() -> (w303:refnum<vi>)
        n168 = control-ref of="Jog Left HOM"() -> (w297:refnum<vi>)
        n169 = control-ref of="Focus Steps"() -> (w301:refnum<vi>)
        n170 = control-ref of="Jog Up"() -> (w294:refnum<vi>)
        n171 = control-ref of="Jog Z In"() -> (w292:refnum<vi>)
        n172 = control-ref of="Jog Right"() -> (w296:refnum<vi>)
        n173 = control-ref of="Jog Left"() -> (w298:refnum<vi>)
        n174 = control-ref of="Jog Z Out"() -> (w295:refnum<vi>)
        n175 = control-ref of="Jog Down"() -> (w293:refnum<vi>)
        n176 = property class="Bool"(reference=w294, "Visible"=w291) -> ()  [unwired: 1 in, 2 out]
        n177 = property class="Bool"(reference=w292, "Visible"=w291) -> ()  [unwired: 1 in, 2 out]
        n178 = property class="Bool"(reference=w296, "Visible"=w291) -> ()  [unwired: 1 in, 2 out]
        n179 = property class="Enum (strict)"(reference=w306, "Visible"=w291) -> ()  [unwired: 1 in, 2 out]
        n180 = property class="Enum (strict)"(reference=w307, "Visible"=w302) -> ()  [unwired: 1 in, 2 out]
        n181 = property class="Enum (strict)"(reference=w304, "Visible"=w291) -> ()  [unwired: 1 in, 2 out]
        n182 = property class="Bool"(reference=w298, "Visible"=w291) -> ()  [unwired: 1 in, 2 out]
        n183 = property class="DigNum (strict)"(reference=w303, "Visible"=w289) -> ()  [unwired: 1 in, 2 out]
        n184 = property class="Bool"(reference=w297, "Visible"=w289) -> ()  [unwired: 1 in, 2 out]
        n185 = property class="Bool"(reference=w290, "Visible"=w289) -> ()  [unwired: 1 in, 2 out]
        n186 = property class="Enum (strict)"(reference=w305, "Visible"=w291) -> ()  [unwired: 1 in, 2 out]
        n187 = property class="Bool"(reference=w295, "Visible"=w291) -> ()  [unwired: 1 in, 2 out]
        n188 = property class="Bool"(reference=w293, "Visible"=w291) -> ()  [unwired: 1 in, 2 out]
        n189 = property class="DigNum (strict)"(reference=w301, "Visible"=w291) -> ()  [unwired: 1 in, 2 out]
        n190 = control-ref of="X Pixels"() -> (w299:refnum<vi>)
        n191 = control-ref of="Y Pixels"() -> (w300:refnum<vi>)
        n192 = property class="DigNum (strict)"(reference=w299, "Visible"=w291) -> ()  [unwired: 1 in, 2 out]
        n193 = property class="DigNum (strict)"(reference=w300, "Visible"=w291) -> ()  [unwired: 1 in, 2 out]
      }
      event User Event {
        n194 = event-data() -> ("Scanning Done"=w315:bool, "Axis"=w316:enum16{"X", "Y", "Z", "HOM"})  [unwired: 1 in]
        n195 = Unbundle By Name(w314) -> ("Steps"=w321:u32)
        n196 = local read "Experiment Scan"() -> (w319:i32)
        n197 = Equal?(x=1, y=w319) -> (x = y?=w318:bool)
        n198 = case shown="True" w315 {
          tunnel: w323 -> [w332 w349]
          tunnel: [w331 w344] -> w322
          tunnel: w321 -> [w330 _]
          tunnel: w320 -> [w329 w348]
          tunnel: w318 -> [w327 w346]
          tunnel: w316 -> [w324 w345]
          tunnel: w314 -> [_ w347]
          frame False {
            # "Which Direction? Depends on the Channel"
            n199 = case shown="False" w327 {
              tunnel: [w334 w343] -> w326
              tunnel: [w333 w342] -> w325
              tunnel: w324 -> [w335 _]
              frame False {
                n200 = case shown="\"Y\"" w335 {
                  tunnel: [w337 w339 w341] -> w334
                  tunnel: [w336 w338 w340] -> w333
                  frame "X", Default {
                    n201 = local read "X Scan Direction"() -> (w336:enum16{"Forward", "Backwards"})
                    n202 = local read "X Channel"() -> (w337:i32)
                  }
                  frame "Y" {
                    n203 = local read "Y Scan Direction"() -> (w338:enum16{"Forward", "Backwards"})
                    n204 = local read "Y Channel"() -> (w339:i32)
                  }
                  frame "Z" {
                    n205 = local read "Y Scan Direction"() -> (w340:enum16{"Forward", "Backwards"})
                    n206 = local read "Y Channel"() -> (w341:i32)
                  }
                }
              }
              frame True {
                n207 = local read "Interferometer\nDirection"() -> (w342:enum16{"Forward", "Backwards"})
                n208 = local read "HOM Channel"() -> (w343:i32)
              }
            }
            n209 = call "Send MoveBySteps.vi"("Direction"=w325, "Steps"=w330, "Message Priority (Normal)"=w326, "error in (no error)"=w332, "Polarity"=enum16{"Positive", "Negative"}."Positive", "Message Enqueuer"=w329) -> ("error out"=w331:errorcluster)  [unwired: 4 in, 1 out]
          }
          frame True {
            n210 = case shown="False" w346 {
              tunnel: w345 -> [w379 _]
              tunnel: w347 -> [w383 _]
              tunnel: [w382 0 ("Home 2")] -> w358
              tunnel: [w381 w395] -> w357
              tunnel: [w380 TRUE] -> w353
              frame False {
                n211 = case shown="\"Y\"" w379 {
                  tunnel: w383 -> [w387 w392]
                  tunnel: [w386 w390] -> w382
                  tunnel: [w384 w388] -> w381
                  tunnel: [TRUE w389] -> w380
                  frame "X", Default {
                    n212 = Unbundle By Name(w387) -> ("Home 1"=w386:i32)
                    n213 = local read "X Channel"() -> (w384:i32)
                  }
                  frame "Y" {
                    n214 = Unbundle By Name(w392) -> ("Home 2"=w390:i32)
                    n215 = local read "Position Z"() -> (w391:i32)
                    n216 = local read "Y Channel"() -> (w388:i32)
                    n217 = Not Equal?(x=w391, y=w390) -> (x != y?=w389:bool)
                  }
                }
              }
              frame True {
                n218 = local read "HOM Channel"() -> (w395:i32)
              }
            }
            n219 = Bundle By Name(cluster=w347, "Going Home?"=TRUE) -> (w351:T4)
            n220 = Unbundle By Name(w351) -> ("Selected Motor"=w356:enum16{"KIM", "Stepper Motors"}, "Scan Segments"=w355:u32, "Steps"=w354:u32)
            n221 = Multiply(x=w355, y=w354) -> ()  [unwired: 1 out]
            n222 = case shown="\"KIM\", Default" w356 {
              tunnel: w348 -> [w365 w378]
              tunnel: w358 -> [w364 w373]
              tunnel: TRUE ("Home?") -> [w363 w376]
              tunnel: [w362 w374] -> w344
              tunnel: w349 -> [w361 w375]
              tunnel: w357 -> [w360 w377]
              tunnel: w353 -> [w359 _]
              frame "KIM", Default {
                n223 = case shown="True" w359 {
                  tunnel: w365 -> [_ w372]
                  tunnel: w364 -> [_ w371]
                  tunnel: w363 -> [_ w367]
                  tunnel: [w366 w370] -> w362
                  tunnel: w361 -> [w366 w369]
                  tunnel: w360 -> [_ w368]
                  frame False {
                  }
                  frame True {
                    n224 = call "Send Goto.vi"("Home?"=w367, "error in (no error)"=w369, "channel"=w368, "New Position"=w371, "Message Enqueuer"=w372) -> ("error out"=w370:errorcluster)  [unwired: 5 in, 1 out]
                  }
                }
              }
              frame "Stepper Motors" {
                n225 = call "Send Goto.vi"("Home?"=w376, "error in (no error)"=w375, "channel"=w377, "New Position"=w373, "Message Enqueuer"=w378) -> ("error out"=w374:errorcluster)  [unwired: 5 in, 1 out]
              }
            }
          }
        }
      }
      event User Event {
        n226 = event-data() -> ("CH1 Pos"=w407:i32, "CH2 Pos"=w406:i32, "CH3 Pos"=w405:i32, "CH4 Pos"=w404:i32, "Home?"=w400:bool)  [unwired: 1 in]
        n227 = local write "Position Y"(w405) -> ()
        n228 = local write "Position HOM"(w404) -> ()
        n229 = local write "Position X"(w407) -> ()
        n230 = local write "Position Z"(w406) -> ()
        n231 = Unbundle By Name(w403) -> ("Going Home?"=w399:bool, "Scanning Instrument"=w397:bool, "Scanning Motor"=w396:bool)
        n232 = Bundle By Name(cluster=w403, "Going Home?"=FALSE) -> (w401:T4)
        n233 = Or(x=w396, y=w397) -> (x .or. y?=w398:bool)
        n234 = case shown="False" w398 {
          tunnel: w411 -> [_ w420]
          tunnel: w409 -> [w415 w419]
          tunnel: [w412 w418] -> w410
          tunnel: w401 -> [w413 w416]
          tunnel: [w413 w416] -> w408
          tunnel: w399 -> [_ _]
          tunnel: w400 -> [_ w417]
          frame False {
            n235 = property on="Scan" class="Bool"(error in=w415, "DisabledEnum"=T5."Enabled" ("Disabled")) -> (error out=w412:errorcluster)  [unwired: 1 in, 1 out]
          }
          frame True {
            n236 = call "Send StageMoved.vi"("error in (no error)"=w419, "Home?"=w417, "Message Enqueuer"=w420) -> ("error out"=w418:errorcluster)  [unwired: 7 in, 1 out]
          }
        }
      }
      event User Event {
        w427 = T5."Disabled and Grayed Out" ("Disabled")
        w422 = FALSE ("Scanning")
        n237 = event-data() -> ()  [unwired: 1 in, 3 out]
        n238 = local write "Scanning"(FALSE ("Scanning")) -> ()
        n239 = Bundle By Name(cluster=w437, "Scanning Motor"=w422, "Scanning Instrument"=w422) -> (w436:T4)
        n240 = local read "Experiment Scan"() -> (w426:i32)
        n241 = case shown="1" w426 {
          tunnel: w425 -> [_ w443]
          tunnel: w424 -> [w440 w442]
          tunnel: [w440 w441] -> w423
          frame 0, Default {
          }
          frame 1 {
            n242 = call "Send JX_GoHome.vi"("error in (no error)"=w442, "Message Enqueuer"=w443) -> ("error out"=w441:errorcluster)  [unwired: 8 in, 1 out]
          }
        }
        n243 = control-ref of="Init motor"() -> (w433:refnum<vi>)
        n244 = property class="VI"() -> ("Panel"=w439:refnum<vi>)  [unwired: 2 in, 2 out]
        n245 = control-ref of="Address"() -> (w435:refnum<vi>)
        n246 = control-ref of="Control"() -> (w434:refnum<vi>)
        n247 = property class="Enum (strict)"(reference=w434, "DisabledEnum"=w427) -> (error out=w432:errorcluster)  [unwired: 1 in, 1 out]
        n248 = property class="Bool"(reference=w433, "DisabledEnum"=w427) -> (error out=w430:errorcluster)  [unwired: 1 in, 1 out]
        n249 = call "EnableControls.vi"("error in (no error)"=w423, "Disabled"=T5."Enabled", "Panel in"=w439) -> ("error out"=w429:errorcluster)  [unwired: 8 in]
        n250 = property class="Str"(reference=w435, "DisabledEnum"=w427) -> (error out=w431:errorcluster)  [unwired: 1 in, 1 out]
        n251 = Merge Errors(w432, w431, w430, w429) -> (w428:errorcluster)
      }
      event User Event {
        n252 = event-data() -> ()  [unwired: 1 in, 3 out]
      }
      event "Exit": Value Change {
        n253 = event-data() -> ()  [unwired: 1 in, 3 out]
        n254 = call <vilib>:"Send Normal Stop.vi"("Message Enqueuer"=w449) -> ()  [unwired: 10 in, 1 out]
        n255 = call <vilib>:"Send Normal Stop.vi"("Message Enqueuer"=w450) -> ()  [unwired: 10 in, 1 out]
      }
      event Panel Close? {
        n256 = event-data() -> ()  [unwired: 1 in, 3 out]
        n257 = call <vilib>:"Send Normal Stop.vi"("Message Enqueuer"=w453) -> ()  [unwired: 10 in, 1 out]
        n258 = call <vilib>:"Send Normal Stop.vi"("Message Enqueuer"=w454) -> ()  [unwired: 10 in, 1 out]
        n259 = event-data("Discard?"=TRUE) -> ()  [unwired: 1 in, 1 out]
      }
    }
  }
  n260 = Unregister For Events(event registration refnum=w13) -> ()  [unwired: 1 in, 1 out]
